vi "WPI_PotentiometerGetNormalized.vi"(8 "error in":errorcluster, 11 "PotDevRef":T1) -> (0 "error out":errorcluster, 2 "Normalized Value":dbl, 3 "PotDevRef":T1)   [LabVIEW 2017]
doc: "Returns the Normalized Value from the potentiometer. Normalization is the result of comparing the potentiometer return voltage to the 5 Volt Rail voltage of the controller that is used to power the potentiometer. This assures that the Normalized Value is from 0 to 1.\n\n\nThis software is licensed. Open the labview\\readme\\WPI Robotics Library Open Source License.txt file for more information."
uses:
  <vilib>/Rock Robotics/WPI/Potentiometer/WPI_PotentiometerDevRef.ctl
  <vilib>/Rock Robotics/SystemInterfaces/AI/FPGA_AIChannel.ctl
  <vilib>/Rock Robotics/WPI/AnalogChannel/WPI_AnalogChannelDevRef.ctl
  <vilib>/Rock Robotics/WPI/Power/WPI_Power Get 5Volt Rail Voltage and Current.vi
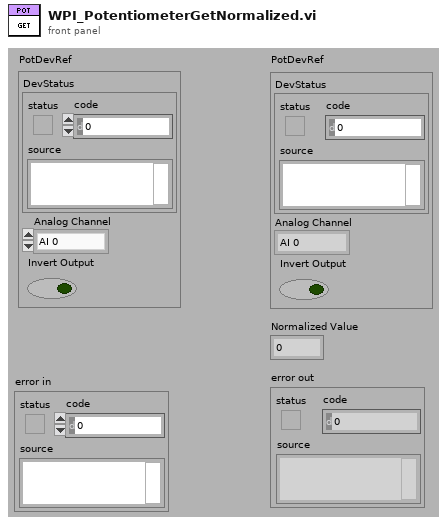
[diagram p1: front panel]
types:
  T1 = typedef "WPI_PotentiometerDevRef.ctl" = cluster{"DevStatus":errorcluster, "Analog Channel":T2, "Invert Output":bool}
  T2 = typedef "FPGA_AIChannel.ctl" = enum8{"AI 0", "AI 1", "AI 2", "AI 3", "AI MXP 0", "AI MXP 1", "AI MXP 2", "AI MXP 3", "Invalid"}
  T3 = typedef "WPI_AnalogChannelDevRef.ctl" = cluster{"DevStatus":errorcluster, "Analog Channel":T2}
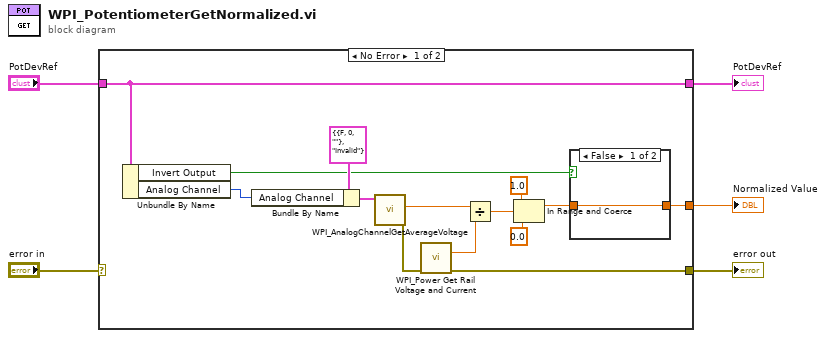
[diagram p0: block diagram]
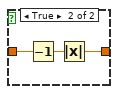
[diagram p2: hidden frame]
diagram:
  n1 = case shown="No Error" "error in" {
    selector: "error in" -> [_ w25]
    tunnel: "PotDevRef" -> [w13 w24]
    tunnel: [w15 w25] -> w4
    tunnel: [w8 _] -> w2
    tunnel: [w13 w24] -> w1
    frame No Error {
      n2 = Unbundle By Name(w13) -> ("Invert Output"=w7:bool, "Analog Channel"=w18:T2)
      n3 = Bundle By Name(cluster=T3 {"DevStatus"={"status"=FALSE, "code"=0, "source"=""}, "Analog Channel"=enum."Invalid"} ("AIDeviceRef"), "Analog Channel"=w18) -> (w17:T3)
      n4 = call <vilib>:"WPI_AnalogChannelGetAverageVoltage.vi"("AIDeviceRef"=w17) -> ("error out"=w16:errorcluster, "Voltage"=w14:dbl)  [unwired: 8 in, 1 out]
      n5 = call-poly <vilib>:"WPI_Power Get Rail Voltage and Current.vi"("error in"=w16) -> ("5 volt rail voltage (V)"=w6:dbl, "error out"=w15:errorcluster)  [unwired: 12 in, 1 out]
      n6 = Divide(x=w14, y=w6) -> (x/y=w10:dbl)
      n7 = In Range and Coerce(upper limit=1.0, x=w10, lower limit=0.0) -> (coerced(x)=w9:dbl)  [unwired: 1 out]
      n8 = case shown="False" w7 {
        tunnel: w9 -> [w20 w22]
        tunnel: [w20 w21] -> w8
        frame False {
        }
        frame True {
          n9 = Decrement(x=w22) -> (x-1=w23:dbl)
          n10 = Absolute Value(x=w23) -> (abs(x)=w21:dbl)
        }
      }
    }
    frame Error {
    }
  }
  "PotDevRef" <- w1
  "Normalized Value" <- w2
  "error out" <- w4
